vi "Test Static (Global).vi"(8 "error in (no error)":errorcluster, 11 "TestCase in":refnum<class "Verify IMemento.lvclass">) -> (0 "error out":errorcluster, 3 "TestCase out":refnum<class "Verify IMemento.lvclass">)   [LabVIEW 2009, in "Verify IMemento.lvclass"]
uses:
  Verify IMemento.lvclass
  Numeric Test Object/Numeric Test Object.lvclass
  Numeric Test Object/Interface Implementations/IMementoNumeric/IMementoNumeric.lvclass
  Framework Core/Interface Definitions/IMemento/IMemento.lvclass
  Verify IMemento.lvclass/Verify IMemento.ctl
  <vilib>/addons/_JKI Toolkits/VI Tester/TestCase.llb/TestCase.lvclass
  Source/Interfaceable Class/Interfaceable.lvclass
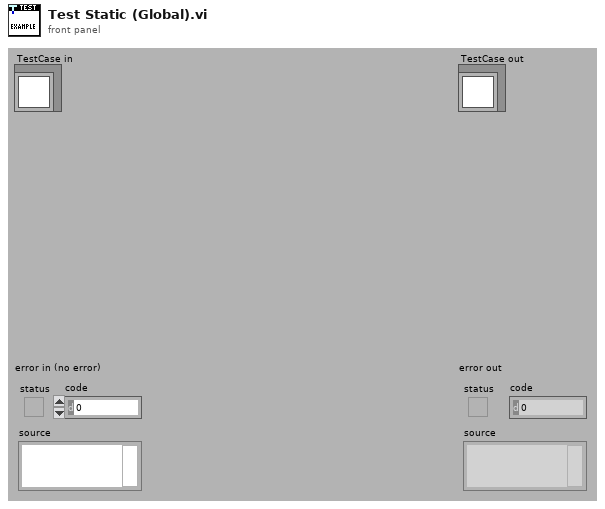
[diagram p1: front panel]
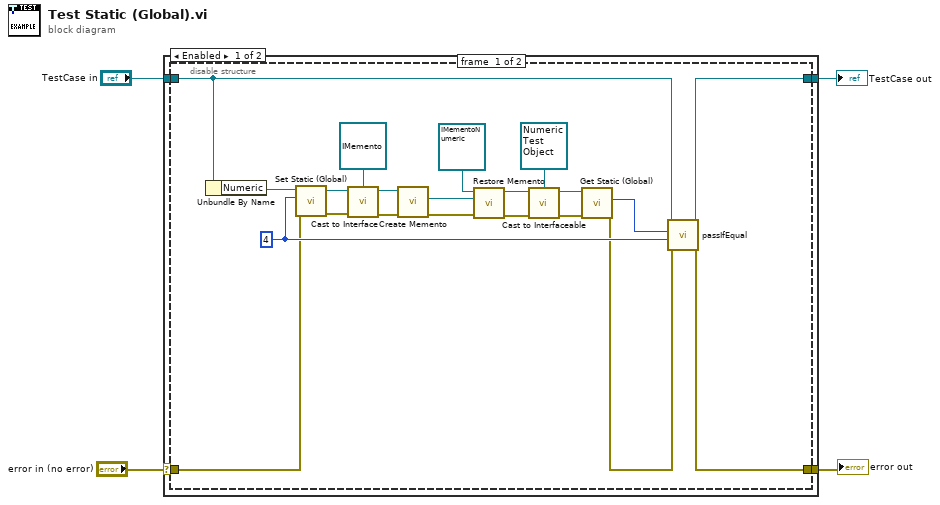
[diagram p0: block diagram]
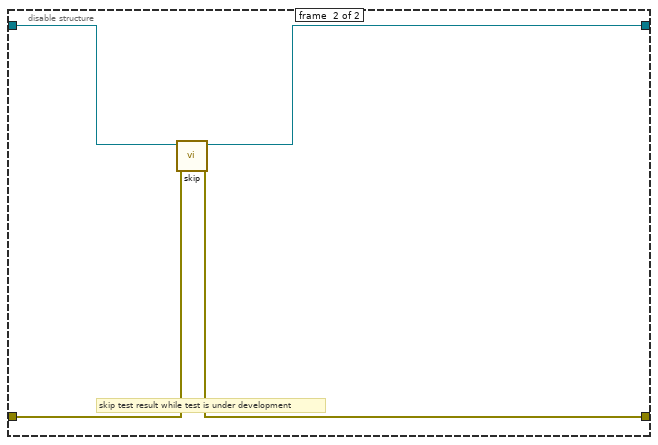
[diagram p2: hidden frame]
diagram:
  n1 = case shown="No Error" "error in (no error)" {
    selector: "error in (no error)" -> [w6 w35]
    tunnel: [w5 w35] -> w3
    tunnel: [w7 w34] -> w1
    tunnel: "TestCase in" -> [w8 w34]
    frame #0 {
      n2 = disable-structure shown="Enabled" {
        disable-tunnel: w8 -> [w27 w33]
        disable-tunnel: [w29 w30] -> w7
        disable-tunnel: w6 -> [w10 w32]
        disable-tunnel: [w28 w31] -> w5
        frame #0 {
          w12 = 4 ("Int")
          n3 = Unbundle By Name(w27) -> ("Numeric"=w26:refnum<class "Numeric Test Object.lvclass">)
          n4 = call-dynamic "Set Static (Global).vi"("error in (no error)"=w10, "Int"=w12, "Numeric in"=w26) -> ("error out"=w24:errorcluster, "Numeric out"=w25:refnum<class "Numeric Test Object.lvclass">)  [unwired: 7 in]
          n5 = call "Cast to Interface.vi"("Target Interface"=refnum<class "IMemento.lvclass"> refnum ("IMemento"), "Interfaceable Object"=w25, "error in (no error)"=w24) -> ("Concrete Interface"=w22:refnum<class "IMemento.lvclass">, "error out"=w21:errorcluster)  [unwired: 5 in]
          n6 = call-dynamic "Create Memento.vi"("error in (no error)"=w21, "IMemento in"=w22) -> ("error out"=w16:errorcluster, "LabVIEW Object"=w20:refnum<class>)  [unwired: 7 in, 1 out]
          n7 = call-dynamic "Restore Memento.vi"("error in (no error)"=w16, "Numeric Memento"=w20, "IMementoNumeric in"=refnum<class "IMementoNumeric.lvclass"> refnum ("IMementoNumeric")) -> ("error out"=w17:errorcluster, "IMementoNumeric out"=w18:refnum<class "IMementoNumeric.lvclass">)  [unwired: 7 in]
          n8 = call "Cast to Interfaceable.vi"("Target Object"=refnum<class "Numeric Test Object.lvclass"> refnum ("Numeric"), "Interface"=w18, "error in (no error)"=w17) -> ("Interfaceable Object"=w14:refnum<class "Numeric Test Object.lvclass">, "error out"=w13:errorcluster)  [unwired: 5 in]
          n9 = call-dynamic "Get Static (Global).vi"("error in (no error)"=w13, "Numeric in"=w14) -> ("error out"=w9:errorcluster, "Int"=w11:i32)  [unwired: 7 in, 1 out]
          n10 = call-dynamic "passIfEqual.vi"("error in (no error)"=w9, "y"=w12, "x"=w11, "TestCase in"=w27) -> ("error out"=w28:errorcluster, "TestCase out"=w29:refnum<class "Verify IMemento.lvclass">)  [unwired: 6 in]
        }
        frame #1 {
          # "skip test result while test is under development"
          n11 = call <vilib>:"skip.vi"("error in (no error)"=w32, "TestCase in"=w33) -> ("error out"=w31:errorcluster, "TestCase out"=w30:refnum<class "Verify IMemento.lvclass">)  [unwired: 8 in]
        }
      }
    }
    frame #1 {
    }
  }
  "error out" <- w3
  "TestCase out" <- w1
